vi "MoveClouds.vi"(8 "error in (no error)":errorcluster, 11 "SnakeGame in":refnum<class "SnakeGame.lvclass">) -> (0 "error out":errorcluster, 3 "SnakeGame out":refnum<class "SnakeGame.lvclass">)   [LabVIEW 2019, in "RT_Game.lvlib" / "SnakeGame.lvclass"]
uses:
  SnakeGame.lvclass
  C:/Users/FreshBob/Dropbox/VIs/myRIO_GameConsole/RT/RT_Game/Game/Game.lvclass
  SnakeGame.lvclass/SnakeGame.ctl
  Game/Game.lvclass/Game.ctl
  GameObject/GameObject.lvclass/GameObject.ctl
  Game/Coordinate.ctl
  GameObject/Read IsActive.vi
  Game/Read Sprites.vi
  Game/Write Sprites.vi
  RT_Sprite/RT_Sprite.lvclass
  C:/Users/FreshBob/Dropbox/VIs/myRIO_GameConsole/RT/RT_Game/GameObject/GameObject.lvclass
  Globals.vi
  RT_Game.lvlib
  GameObject/GameObject.lvclass
  Game/Game.lvclass
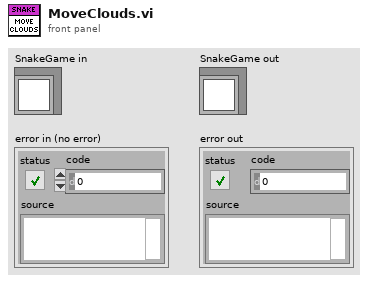
[diagram p1: front panel]
types:
  T1 = typedef "RT_Game.lvlib/Game.lvclass/SpritesCluster.ctl" = cluster{"Sprite1":refnum<class "RT_Sprite.lvclass">, "Sprite2":refnum<class "RT_Sprite.lvclass">, "Sprite3":refnum<class "RT_Sprite.lvclass">}
  T2 = typedef "RT_Game.lvlib/Game.lvclass/Coordinate.ctl" = cluster{"x":dbl, "y":dbl}
  T3 = cluster{"[0]":refnum<class "RT_Sprite.lvclass">, "[1]":refnum<class "RT_Sprite.lvclass">, "[2]":refnum<class "RT_Sprite.lvclass">}
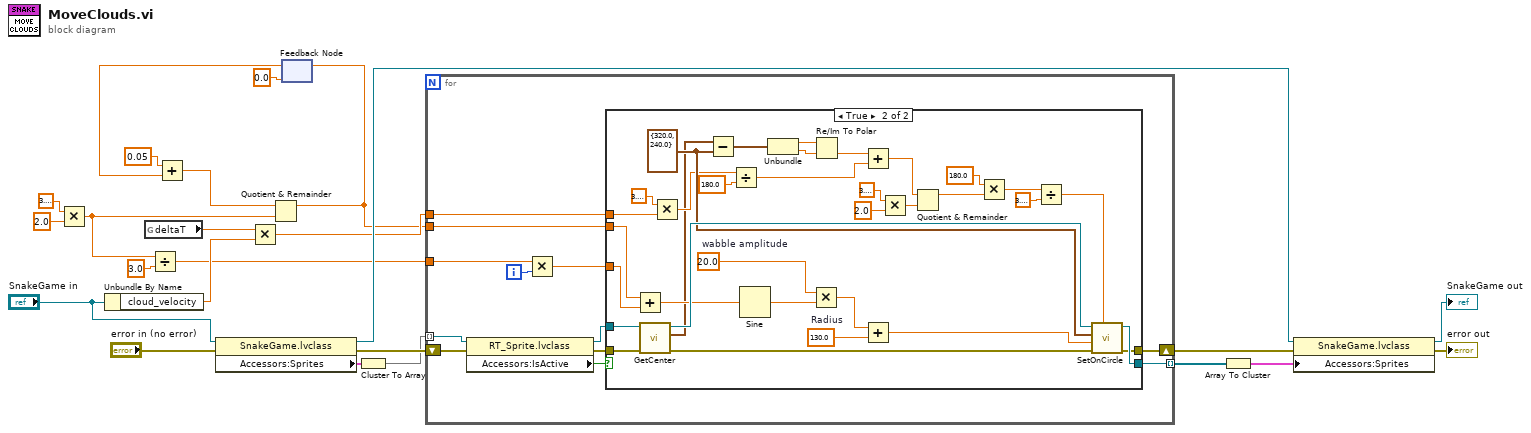
[diagram p0: block diagram]
diagram:
  n1 = Multiply(x=3.141592653589793, y=2.0) -> (x*y=w5:dbl)
  n2 = Unbundle By Name("SnakeGame in") -> ("cloud_velocity"=w13:dbl)
  n3 = global read "Globals.vi" "deltaT"() -> (w14:dbl)
  n4 = Divide(x=w5, y=3.0) -> (x/y=w3:dbl)
  n5 = property class="SnakeGame.lvclass"(reference="SnakeGame in", error in="error in (no error)") -> (reference out=w21:refnum<class "SnakeGame.lvclass">, error out=w23:errorcluster, "Accessors:Sprites"=w19:T1)
  n6 = Multiply(x=w14, y=w13) -> (x*y=w15:dbl)
  n7 = feedback #1(0.0) -> (w11:dbl)
  n8 = Add(x=0.05, y=w11) -> (x+y=w9:dbl)
  n9 = Quotient & Remainder(x=w9, y=w5) -> (x-y*floor(x/y)=w6:dbl)  [unwired: 1 out]
  n10 = feedback-in #1(w6) -> ()
  n11 = Cluster To Array(cluster=w19) -> (array=w1:refnum<class "RT_Sprite.lvclass">[])
  n12 = for {
    tunnel: w1 -> [w27] mode=indexing
    tunnel: [w36] -> w18 mode=indexing
    tunnel: w15 -> [w34]
    shift-right: [w35] -> w17
    shift-left: w23 -> [w29]
    tunnel: w6 -> [w33]
    tunnel: w3 -> [w32]
    i -> [w30]
    n13 = property class="RT_Sprite.lvclass"(reference=w27, error in=w29) -> (reference out=w26:refnum<class "RT_Sprite.lvclass">, error out=w28:errorcluster, "Accessors:IsActive"=w25:bool)
    n14 = Multiply(x=w32, y=w30) -> (x*y=w31:dbl)
    n15 = case shown="True" w25 {
      tunnel: w26 -> [w38 w72]
      tunnel: [w38 w71] -> w36
      tunnel: [w37 w70] -> w35
      tunnel: w34 -> [_ w63]
      tunnel: w33 -> [_ w49]
      tunnel: w31 -> [_ w47]
      tunnel: w28 -> [w37 w42]
      frame False {
      }
      frame True {
        w43 = 20.0  # wabble amplitude
        w46 = 130.0  # Radius
        w68 = T2 {"x"=320.0, "y"=240.0} ("Center")
        n16 = Add(x=w49, y=w47) -> (x+y=w48:dbl)
        n17 = call "GetCenter.vi"("error in (no error)"=w42, "GameObject in"=w72) -> ("error out"=w41:errorcluster, "center_pos"=w40:T2, "GameObject out"=w69:refnum<class "RT_Sprite.lvclass">)  [unwired: 7 in]
        n18 = Multiply(x=3.141592653589793, y=w63) -> (x*y=w61:dbl)
        n19 = Subtract(x=w40, y=w68) -> (x-y=w67:T2)
        n20 = Divide(x=w61, y=180.0) -> (x/y=w59:dbl)
        n21 = Sine(x=w48) -> (sin(x)=w45:dbl)
        n22 = Unbundle(w67) -> ("x"=w66:dbl, "y"=w65:dbl)
        n23 = Multiply(x=w43, y=w45) -> (x*y=w44:dbl)
        n24 = Re/Im To Polar(2:w65, 3:w66) -> (0:w64:dbl)  [unwired: 1 out]
        n25 = Add(x=w64, y=w59) -> (x+y=w58:dbl)
        n26 = Add(x=w44, y=w46) -> (x+y=w39:dbl)
        n27 = Multiply(x=3.141592653589793, y=2.0) -> (x*y=w56:dbl)
        n28 = Quotient & Remainder(x=w58, y=w56) -> (x-y*floor(x/y)=w54:dbl)  [unwired: 1 out]
        n29 = Multiply(x=180.0, y=w54) -> (x*y=w53:dbl)
        n30 = Divide(x=w53, y=3.141592653589793) -> (x/y=w51:dbl)
        n31 = call "SetOnCircle.vi"("angle (deg)"=w51, "error in (no error)"=w41, "Radius"=w39, "Center"=w68, "GameObject in"=w69) -> ("error out"=w70:errorcluster, "GameObject out"=w71:refnum<class "RT_Sprite.lvclass">)  [unwired: 5 in]
      }
    }
  }
  n32 = Array To Cluster(array=w18) -> (cluster=w2:T3)
  n33 = property class="SnakeGame.lvclass"(reference=w21, error in=w17, "Accessors:Sprites"=w2) -> (reference out=→"SnakeGame out":refnum<class "SnakeGame.lvclass">, error out=→"error out":errorcluster)
